vi "read eip channels.vi"(8 "error in":errorcluster, 11 "EthernetIP configuration in":refnum<class "EIP Tags Configuration.lvclass">) -> (0 "error out":errorcluster, 2 "channels":refnum<class "EIP Tags Channel.lvclass">[](array[class]), 3 "EthernetIP configuration out":refnum<class "EIP Tags Configuration.lvclass">)   [LabVIEW 2013, in "EIP Tags Configuration.lvclass"]
uses:
  EIP Tags Configuration.lvclass
  channel/EIP Tags Channel.lvclass
  EIP Tags Configuration.lvclass/EIP Tags Configuration.ctl
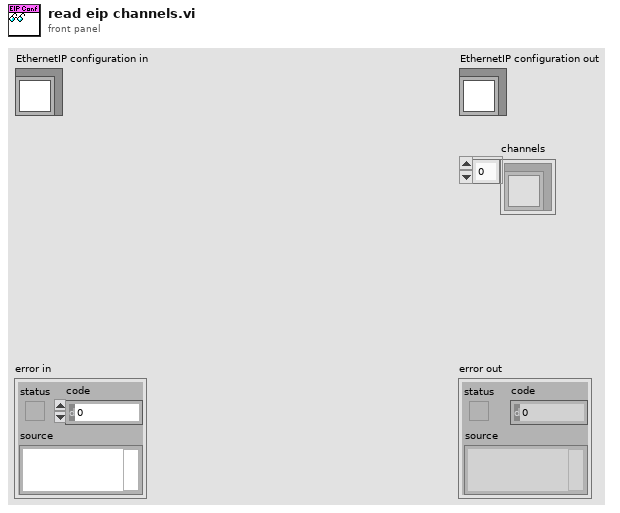
[diagram p1: front panel]
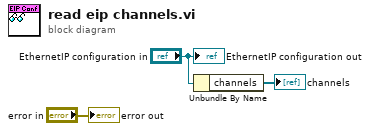
[diagram p0: block diagram]
diagram:
  n1 = Unbundle By Name("EthernetIP configuration in") -> ("channels"=→"channels":refnum<class "EIP Tags Channel.lvclass">[])
  "error out" <- "error in"
  "EthernetIP configuration out" <- "EthernetIP configuration in"
